vi "Get Logic Status (multiple).vi"(8 "error in (no error)":errorcluster, 10 "Array of Pin #":u8[](array[numeric]), 11 "LogicIO in":refnum<class "LogicIO.lvclass">) -> (0 "error out":errorcluster, 2 "Array of Logic Statuses":bool[](array[boolean]), 3 "LogicIO out":refnum<class "LogicIO.lvclass">)   [LabVIEW 2016, in "Hardware.lvlib" / "LogicIO.lvlib" / "LogicIO.lvclass"]
uses:
  <userlib>/Common Components/Hardware/LogicIO/LogicIO/LogicIO.lvclass
  <vilib>/Utility/error.llb/Error Cluster From Error Code.vi
  <vilib>/ErrorRing/Error Ring.xnode
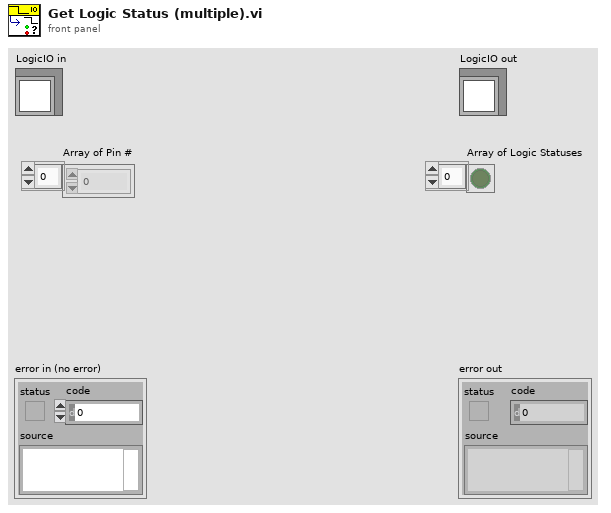
[diagram p1: front panel]
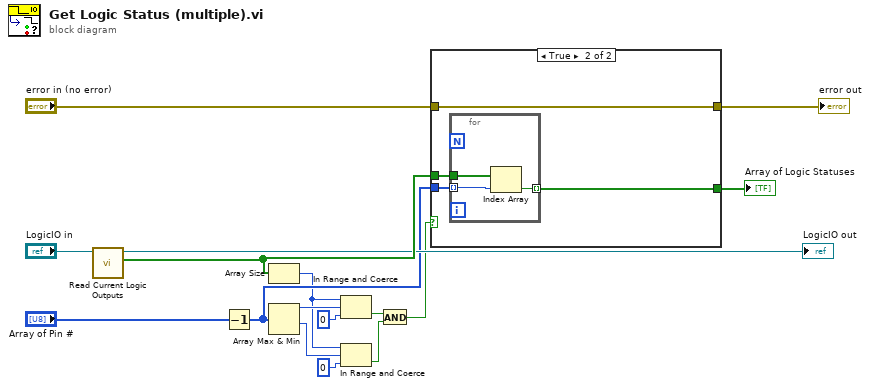
[diagram p0: block diagram]
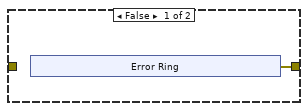
[diagram p2: hidden frame]
diagram:
  n1 = call <userlib>:"Read Current Logic Outputs.vi"("LogicIO in"="LogicIO in") -> ("Current Logic Outputs"=w12:bool[], "LogicIO out"=→"LogicIO out":refnum<class "LogicIO.lvclass">)  [unwired: 9 in]
  n2 = Decrement(x="Array of Pin #") -> (x-1=w2:u8[])
  n3 = Array Size(array=w12) -> (size(s)=w1:i32)
  n4 = Array Max & Min(array=w2) -> (max value=w6:u8, min value=w7:u8)  [unwired: 2 out]
  n5 = In Range and Coerce(upper limit=w1, x=w6, lower limit=0) -> (In Range?=w5:bool)  [unwired: 1 out]
  n6 = In Range and Coerce(upper limit=w1, x=w7, lower limit=0) -> (In Range?=w4:bool)  [unwired: 1 out]
  n7 = And(x=w5, y=w4) -> (x .and. y?=w3:bool)
  n8 = case shown="True" w3 {
    tunnel: w12 -> [_ w22]
    tunnel: w2 -> [_ w25]
    tunnel: [_ w24] -> w14
    tunnel: "error in (no error)" -> [_ w23]
    tunnel: [w17 w23] -> w15
    frame False {
      n9 = xnode "Error Ring"() -> ("error out"=w17:errorcluster)
    }
    frame True {
      n10 = for {
        tunnel: w22 -> [w28]
        tunnel: w25 -> [w27] mode=indexing
        tunnel: [w26] -> w24 mode=indexing
        n11 = Index Array(array=w28, index=w27) -> (element=w26:bool)
      }
    }
  }
  "error out" <- w15
  "Array of Logic Statuses" <- w14
